vi "Data Replay DBLs to Waveform.vi"(9 "display two rotations? (F)":bool, 10 "CycleAngle?":T1, 11 "Data":dbl[](array[numeric])) -> (3 "waveform":waveform(dbl))   [LabVIEW 2011, in "Engine Sim System Explorer.lvlib"]
uses:
  Engine Sim System Explorer.lvlib
  TypeDefs/AngleReference.ctl
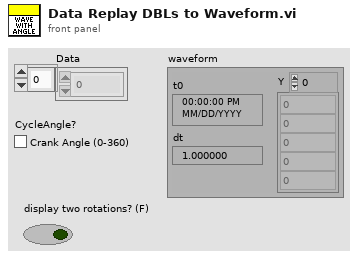
[diagram p1: front panel]
types:
  T1 = typedef "Engine Sim System Explorer.lvlib/AngleReference.ctl" = bool
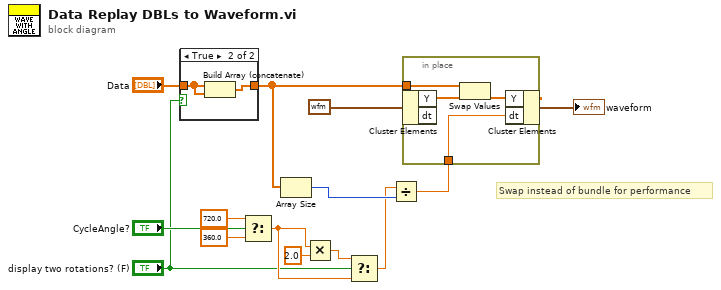
[diagram p0: block diagram]
diagram:
  # "Swap instead of bundle for performance"
  n1 = case shown="True" "display two rotations? (F)" {
    tunnel: [w15 w17] -> w3
    tunnel: "Data" -> [w15 w16]
    frame False {
    }
    frame True {
      n2 = Build Array (concatenate)(w16, w16) -> (w17:dbl[])
    }
  }
  n3 = Select(t=720.0, s="CycleAngle?", f=360.0) -> (s? t:f=w5:dbl)
  n4 = Array Size(array=w3) -> (size(s)=w9:i32)
  n5 = Multiply(x=w5, y=2.0) -> (x*y=w7:dbl)
  n6 = Select(t=w7, s="display two rotations? (F)", f=w5) -> (s? t:f=w4:dbl)
  n7 = Divide(x=w4, y=w9) -> (x/y=w13:dbl)
  n8 = in-place {
    in-place-border: w3 -> [w20]
    in-place-border: w13 -> [w18]
    n9 = in-place-cluster #1(waveform(dbl) {"t0"=timestamp(0 s since 1904-01-01), "dt"=1.0, "Y"=[]} ("waveform")) -> ("Y"=w21:dbl[])  [unwired: 1 out]
    n10 = Swap Values(12:w20, 14:w21) -> (3:w19:dbl[])  [unwired: 1 in, 1 out]
    n11 = in-place-cluster #1("Y"=w19, "dt"=w18) -> (→"waveform":waveform(dbl))
  }
